vi "Stop Core.vi"(10 "final error code":i32, 11 "Cooler UI with Events in":refnum<class "Cooler UI with Events.lvclass">) -> (3 "Cooler UI with Events out":refnum<class "Cooler UI with Events.lvclass">)   [LabVIEW 2012, in "Cooler UI.lvlib" / "Cooler UI with Events.lvclass"]
doc: "In override VIs of Stop Core.vi, an actor should invoke any code needed to stop all the parallel processes that it created during its run. This includes any nested actors that it created and any other asynchronously running VIs, such as a Time-Delated Message. It may also include all parallel loops in its Actor Core, although it is acceptable to stop those using a local signal on the Actor Core block diagram that is raised after the Call Parent Node finishes. \n\nThe <b>final error code</b> input tells the actor what error was set when this actor quit. Zero means there was no error. You can use this to decide whether this should be treated as a Normal Stop or an Emergency Stop for the purposes of signaling other actors. In general, any non-zero value should be treated as an Emergency Stop, though a given actor is free to choose other policies. Note that the particular error code 1608 indicates that this actor was itself stopped by an Emergency Stop and should pass that along."
uses:
  Cooler UI with Events.lvclass
  <vilib>/ActorFramework/Actor/Actor.lvclass
  Cooler UI with Events.lvclass/Cooler UI with Events.ctl
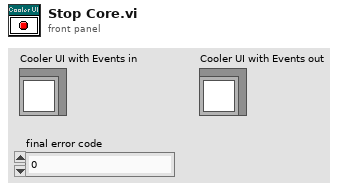
[diagram p1: front panel]
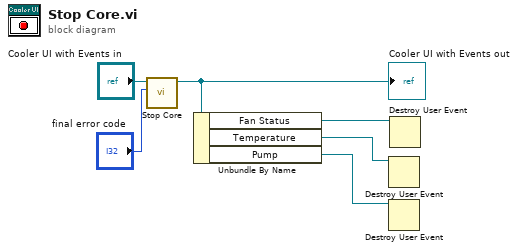
[diagram p0: block diagram]
diagram:
  n1 = call-parent "Stop Core.vi"("final error code"="final error code", "Actor in"="Cooler UI with Events in") -> ("Actor out"=w4:refnum<class "Cooler UI with Events.lvclass">)  [unwired: 9 in]
  "Cooler UI with Events out" <- w4
  n2 = Unbundle By Name(w4) -> ("Fan Status"=w3:refnum<user-event>, "Temperature"=w2:refnum<user-event>, "Pump"=w1:refnum<user-event>)
  n3 = Destroy User Event(user event=w2) -> ()  [unwired: 1 in, 1 out]
  n4 = Destroy User Event(user event=w1) -> ()  [unwired: 1 in, 1 out]
  n5 = Destroy User Event(user event=w3) -> ()  [unwired: 1 in, 1 out]
